vi "login_bage.vi"() -> ()   [LabVIEW 2016]
uses:
  <vilib>/Utility/config.llb/Write Key (String).vi
  <vilib>/Utility/config.llb/Read Key (String).vi
  <vilib>/Utility/file.llb/Write Delimited Spreadsheet (string).vi
  <vilib>/Utility/config.llb/NI_LVConfig.lvlib
panel:
  in  "Choose the CSV file here":path
  in  "Tab Control":enum32{"SIGN IN", "SIGN UP"}(tab)
  in  "Cluster":T1
  in  "Cluster 2":T2
  in  "Choose the INI  file here":path
  out "WARNING":bool
  out "number":dbl[](array[numeric])
  out "Array":string[](array[string])
  # "LOGIN PAGE"
  # "SIGN IN"
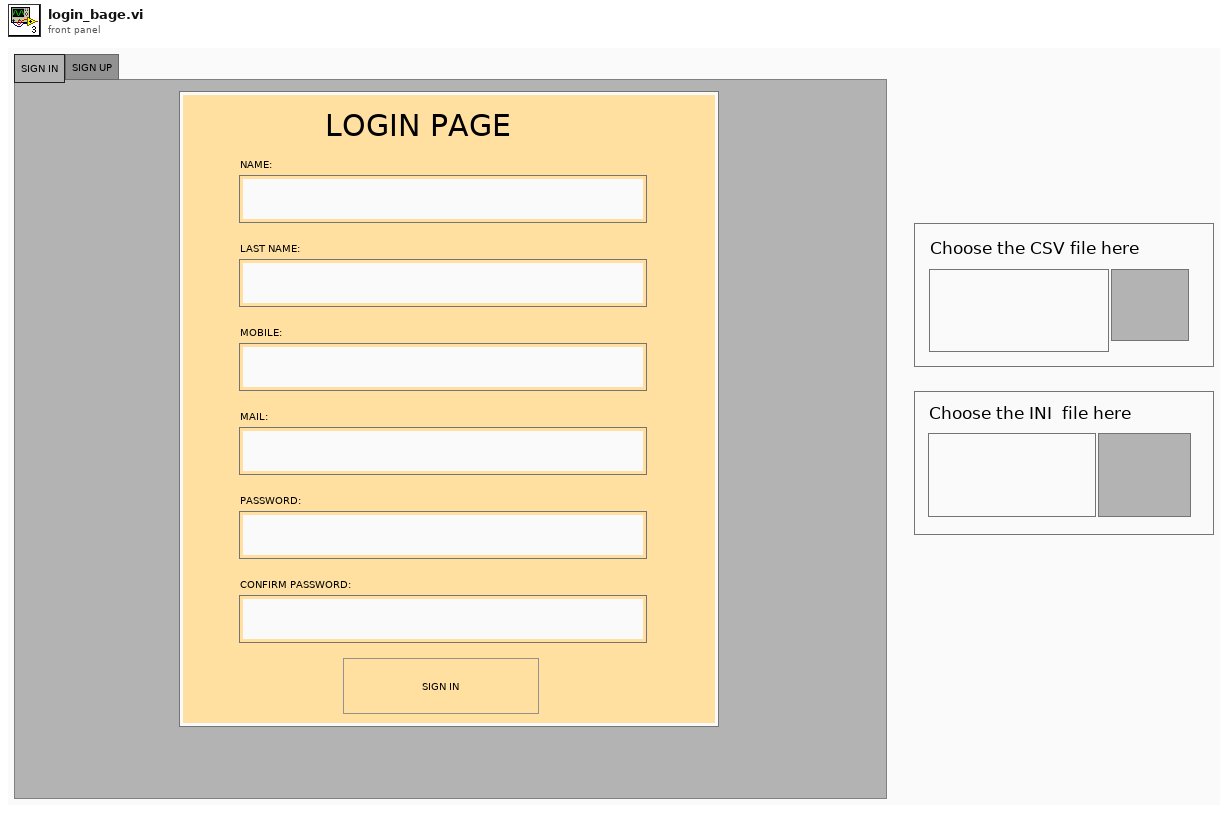
[diagram p1: front panel]
types:
  T1 = cluster{"NAME:":string, "LAST NAME:":string, "MOBILE:":string, "MAIL: ":string, "Boolean":bool, "PASSWORD:":string, "CONFIRM PASSWORD:":string}
  T2 = cluster{"USER NAME:":string, "PASSWORD:":string, "sign":bool}
  T3 = typedef "NI_LVConfig.lvlib/Config Data RefNum.ctl" = refnum<k1>
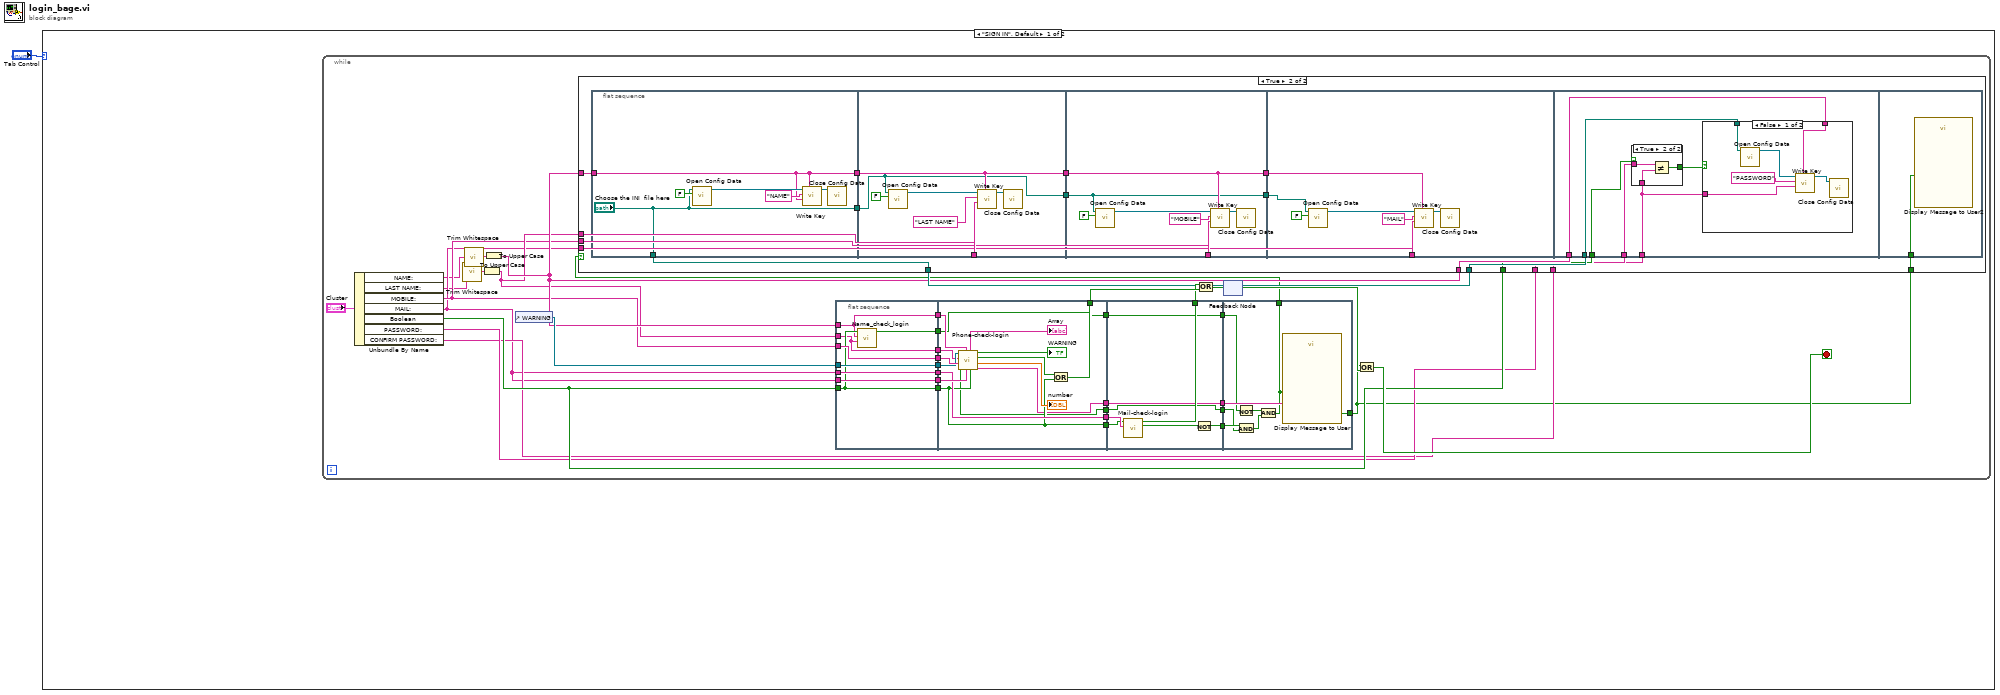
[diagram p0: block diagram]
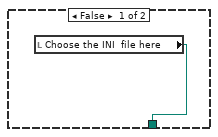
[diagram p2: hidden frame]
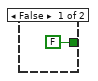
[diagram p3: hidden frame]
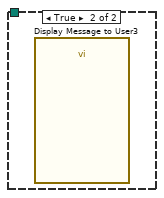
[diagram p4: hidden frame]
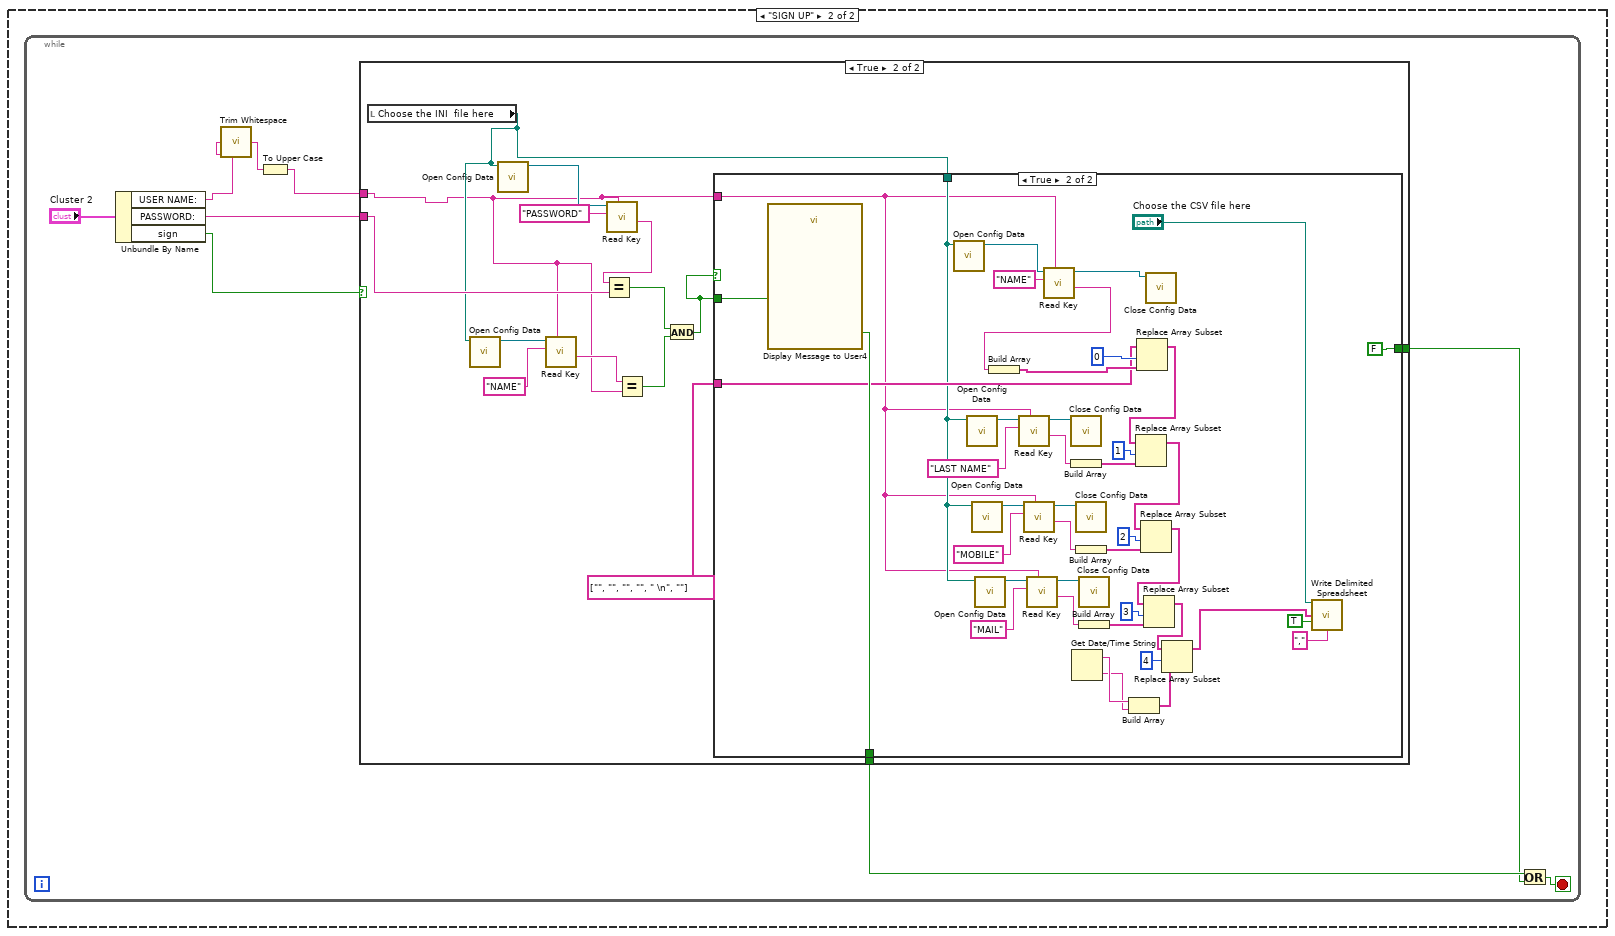
[diagram p5: hidden frame]
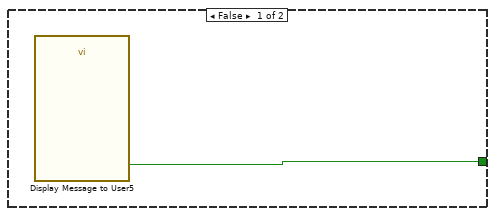
[diagram p7: hidden frame]
diagram:
  n1 = case shown="\"SIGN IN\", Default" "Tab Control" {
    frame "SIGN IN", Default {
      n2 = while {
        stop <- w17 stop-if-true
        n3 = Unbundle By Name("Cluster") -> ("NAME:"=w6:string, "LAST NAME:"=w4:string, "MOBILE:"=w9:string, "MAIL:"=w8:string, "Boolean"=w14:bool, "PASSWORD:"=w13:string, "CONFIRM PASSWORD:"=w12:string)
        n4 = call <vilib>:"Trim Whitespace.vi"("string"=w4) -> ("trimmed string"=w3:string)  [unwired: 1 in]
        n5 = call <vilib>:"Trim Whitespace.vi"("string"=w6) -> ("trimmed string"=w5:string)  [unwired: 1 in]
        n6 = To Upper Case(1:w3) -> (0:w10:string)
        n7 = To Upper Case(1:w5) -> (0:w11:string)
        n8 = control-ref of="WARNING"() -> (w38:refnum<vi>)
        n9 = flat-sequence {
          tunnel: w8 -> [w106]
          tunnel: w38 -> [w107]
          tunnel: w14 -> [w105]
          tunnel: w8 -> [w108]
          tunnel: w9 -> [w109]
          tunnel: w10 -> [w103]
          tunnel: w11 -> [w104]
          tunnel: [w104] -> w28
          tunnel: [w103] -> w27
          tunnel: [w109] -> w26
          tunnel: [w108] -> w25
          tunnel: [w105] -> w24
          tunnel: [w107] -> w23
          tunnel: [w106] -> w22
          tunnel: [w102] -> w21
          tunnel: [w117] -> w36
          tunnel: [w116] -> w37
          tunnel: [w115] -> w34
          tunnel: [w114] -> w33
          tunnel: [w113] -> w32
          tunnel: w28 -> [w112]
          tunnel: w27 -> [w111]
          tunnel: w26 -> [w124]
          tunnel: w25 -> [w123]
          tunnel: w24 -> [w115]
          tunnel: w23 -> [w121]
          tunnel: w22 -> [w116]
          tunnel: w21 -> [w110]
          tunnel: [w110] -> w20
          tunnel: w37 -> [w132]
          tunnel: [w131] -> w35
          tunnel: w34 -> [w126]
          tunnel: [w130] -> w31
          tunnel: w33 -> [w130]
          tunnel: [w129] -> w30
          tunnel: w32 -> [w129]
          tunnel: [w127] -> w29
          tunnel: w20 -> [w125]
          tunnel: [w125] -> w19
          tunnel: w31 -> [w137]
          tunnel: w30 -> [w136]
          tunnel: w29 -> [w138]
          tunnel: w19 -> [w135]
          tunnel: [w134] -> w7
          tunnel: [w133] -> w2
          frame #0 {
            n10 = call "Name_check_login.vi"("LAST NAME:"=w103, "NAME:"=w104, "Boolean"=w105) -> ("OK"=w102:bool)  [unwired: 8 in]
          }
          frame #1 {
            n11 = call "Phone-check-login.vi"("Boolean"=w115, "MAIL:"=w123, "NAME:"=w112, "MOBILE:"=w124, "LAST NAME:"=w111, "Boolean in"=w121) -> ("Info_data"=w113:string, "number"=→"number":dbl[], "Boolean 2"=w122:bool, "WARNING"=→"WARNING":bool, "Array"=→"Array":string[], "sts"=w114:bool)
            n12 = Or(x=w122, y=w115) -> (x .or. y?=w117:bool)
          }
          frame #2 {
            n13 = call "Mail-check-login.vi"("MAIL:"=w132, "Boolean"=w126) -> ("OK2"=w128:bool, "OK"=w131:bool)  [unwired: 8 in]
            n14 = Not(x=w128) -> (.not. x?=w127:bool)
          }
          frame #3 {
            n15 = Not(x=w135) -> (.not. x?=w140:bool)
            n16 = And(x=w138, y=w137) -> (x .and. y?=w139:bool)
            n17 = And(x=w140, y=w139) -> (x .and. y?=w133:bool)
            n18 = call "Display Message to User"("Enable"=w133, "Message"=w136) -> ("OK"=w134:bool)  [unwired: 8 in, 1 out]
          }
        }
        n19 = Or(x=w35, y=w36) -> (x .or. y?=w18:bool)
        n20 = feedback #1() -> (w15:path)  [unwired: 1 in]
        n21 = case shown="True" w2 {
          tunnel: w11 -> [_ w57]
          tunnel: w10 -> [_ w53]
          tunnel: w9 -> [_ w52]
          tunnel: w8 -> [_ w51]
          tunnel: [w40 w47] -> w16
          tunnel: w15 -> [_ w46]
          tunnel: w11 -> [_ w45]
          tunnel: w14 -> [_ w44]
          tunnel: w13 -> [_ w43]
          tunnel: w12 -> [_ w42]
          tunnel: w7 -> [_ w41]
          frame False {
            n22 = local read "Choose the INI  file here"() -> (w40:path)
          }
          frame True {
            n23 = flat-sequence {
              tunnel: w57 -> [w58]
              tunnel: [w58] -> w56
              tunnel: ["Choose the INI  file here"] -> w50
              tunnel: ["Choose the INI  file here"] -> w47
              tunnel: w56 -> [w69]
              tunnel: [w69] -> w55
              tunnel: w53 -> [w64]
              tunnel: w50 -> [w65]
              tunnel: [w65] -> w49
              tunnel: w55 -> [w76]
              tunnel: [w76] -> w54
              tunnel: w52 -> [w71]
              tunnel: w49 -> [w72]
              tunnel: [w72] -> w48
              tunnel: w54 -> [w82]
              tunnel: w51 -> [w78]
              tunnel: w48 -> [w79]
              tunnel: w46 -> [w90]
              tunnel: w45 -> [w89]
              tunnel: w44 -> [w88]
              tunnel: w43 -> [w87]
              tunnel: w42 -> [w86]
              tunnel: w41 -> [w101]
              frame #0 {
                n24 = call <vilib>:"Open Config Data.vi"("create file if necessary (T)"=FALSE, "configuration file path"="Choose the INI  file here") -> ("refnum"=w60:T3)  [unwired: 7 in, 2 out]
                n25 = call-poly <vilib>:"Write Key.vi"("section"=w58, "value"=w58, "key"="NAME", "refnum"=w60) -> ("refnum out"=w62:T3)  [unwired: 5 in, 2 out]
                n26 = call <vilib>:"Close Config Data.vi"("refnum"=w62) -> ()  [unwired: 9 in, 2 out]
              }
              frame #1 {
                n27 = call <vilib>:"Open Config Data.vi"("create file if necessary (T)"=FALSE, "configuration file path"=w65) -> ("refnum"=w66:T3)  [unwired: 7 in, 2 out]
                n28 = call-poly <vilib>:"Write Key.vi"("section"=w69, "value"=w64, "key"="LAST NAME", "refnum"=w66) -> ("refnum out"=w68:T3)  [unwired: 5 in, 2 out]
                n29 = call <vilib>:"Close Config Data.vi"("refnum"=w68) -> ()  [unwired: 9 in, 2 out]
              }
              frame #2 {
                n30 = call <vilib>:"Open Config Data.vi"("create file if necessary (T)"=FALSE, "configuration file path"=w72) -> ("refnum"=w73:T3)  [unwired: 7 in, 2 out]
                n31 = call-poly <vilib>:"Write Key.vi"("section"=w76, "value"=w71, "key"="MOBILE", "refnum"=w73) -> ("refnum out"=w75:T3)  [unwired: 5 in, 2 out]
                n32 = call <vilib>:"Close Config Data.vi"("refnum"=w75) -> ()  [unwired: 9 in, 2 out]
              }
              frame #3 {
                n33 = call <vilib>:"Open Config Data.vi"("create file if necessary (T)"=FALSE, "configuration file path"=w79) -> ("refnum"=w80:T3)  [unwired: 7 in, 2 out]
                n34 = call-poly <vilib>:"Write Key.vi"("section"=w82, "value"=w78, "key"="MAIL", "refnum"=w80) -> ("refnum out"=w84:T3)  [unwired: 5 in, 2 out]
                n35 = call <vilib>:"Close Config Data.vi"("refnum"=w84) -> ()  [unwired: 9 in, 2 out]
              }
              frame #4 {
                n36 = case shown="True" w88 {
                  tunnel: w87 -> [_ w94]
                  tunnel: [FALSE w93] -> w85
                  tunnel: w86 -> [_ w92]
                  frame False {
                  }
                  frame True {
                    n37 = Not Equal?(x=w94, y=w92) -> (x != y?=w93:bool)
                  }
                }
                n38 = case shown="False" w85 {
                  tunnel: w90 -> [w100 _]
                  tunnel: w86 -> [w97 _]
                  tunnel: w89 -> [w95 _]
                  frame False {
                    n39 = call <vilib>:"Open Config Data.vi"("configuration file path"=w100) -> ("refnum"=w99:T3)  [unwired: 8 in, 2 out]
                    n40 = call-poly <vilib>:"Write Key.vi"("section"=w95, "value"=w97, "key"="PASSWORD", "refnum"=w99) -> ("refnum out"=w96:T3)  [unwired: 5 in, 2 out]
                    n41 = call <vilib>:"Close Config Data.vi"("refnum"=w96) -> ()  [unwired: 9 in, 2 out]
                  }
                  frame True {
                    n42 = call "Display Message to User3"() -> ()  [unwired: 10 in, 2 out]
                  }
                }
              }
              frame #5 {
                n43 = call "Display Message to User2"("Enable"=w101) -> ()  [unwired: 9 in, 2 out]
              }
            }
          }
        }
        n44 = feedback-in #1(w16) -> ()
        n45 = Or(x=w7, y=w18) -> (x .or. y?=w17:bool)
      }
    }
    frame "SIGN UP" {
      n46 = while {
        stop <- w148 stop-if-true
        n47 = Unbundle By Name("Cluster 2") -> ("USER NAME:"=w142:string, "PASSWORD:"=w144:string, "sign"=w149:bool)
        n48 = call <vilib>:"Trim Whitespace.vi"("string"=w142) -> ("trimmed string"=w141:string)  [unwired: 1 in]
        n49 = To Upper Case(1:w141) -> (0:w145:string)
        n50 = case shown="True" w149 {
          tunnel: w145 -> [_ w150]
          tunnel: w144 -> [_ w162]
          tunnel: [_ w160] -> w147
          tunnel: [_ w159] -> w146
          frame False {
          }
          frame True {
            n51 = local read "Choose the INI  file here"() -> (w156:path)
            n52 = call <vilib>:"Open Config Data.vi"("configuration file path"=w156) -> ("refnum"=w157:T3)  [unwired: 8 in, 2 out]
            n53 = call <vilib>:"Open Config Data.vi"("configuration file path"=w156) -> ("refnum"=w164:T3)  [unwired: 8 in, 2 out]
            n54 = call-poly <vilib>:"Read Key.vi"("section"=w150, "key"="NAME", "refnum"=w157) -> ("value"=w154:string)  [unwired: 5 in, 3 out]
            n55 = call-poly <vilib>:"Read Key.vi"("section"=w150, "key"="PASSWORD", "refnum"=w164) -> ("value"=w161:string)  [unwired: 5 in, 3 out]
            n56 = Equal?(x=w161, y=w162) -> (x = y?=w152:bool)
            n57 = Equal?(x=w154, y=w150) -> (x = y?=w151:bool)
            n58 = And(x=w152, y=w151) -> (x .and. y?=w153:bool)
            n59 = case shown="True" w153 {
              tunnel: w153 -> [_ w207]
              tunnel: [_ w206] -> w160
              tunnel: [w165 FALSE ("OK")] -> w159
              tunnel: w156 -> [_ w175]
              tunnel: string[] ["", "", "", "", " \n", ""] -> [_ w198]
              tunnel: w150 -> [_ w169]
              frame False {
                n60 = call "Display Message to User5"() -> ("OK"=w165:bool)  [unwired: 10 in, 1 out]
              }
              frame True {
                n61 = call "Display Message to User4"("Enable"=w207) -> ("OK"=w206:bool)  [unwired: 9 in, 1 out]
                n62 = call <vilib>:"Open Config Data.vi"("configuration file path"=w175) -> ("refnum"=w203:T3)  [unwired: 8 in, 2 out]
                n63 = call <vilib>:"Open Config Data.vi"("configuration file path"=w175) -> ("refnum"=w195:T3)  [unwired: 8 in, 2 out]
                n64 = call <vilib>:"Open Config Data.vi"("configuration file path"=w175) -> ("refnum"=w183:T3)  [unwired: 8 in, 2 out]
                n65 = call <vilib>:"Open Config Data.vi"("configuration file path"=w175) -> ("refnum"=w174:T3)  [unwired: 8 in, 2 out]
                n66 = call-poly <vilib>:"Read Key.vi"("section"=w169, "key"="LAST NAME", "refnum"=w195) -> ("value"=w192:string, "refnum out"=w197:T3)  [unwired: 5 in, 2 out]
                n67 = call-poly <vilib>:"Read Key.vi"("section"=w169, "key"="MOBILE", "refnum"=w183) -> ("value"=w186:string, "refnum out"=w181:T3)  [unwired: 5 in, 2 out]
                n68 = call-poly <vilib>:"Read Key.vi"("section"=w169, "key"="MAIL", "refnum"=w174) -> ("value"=w176:string, "refnum out"=w173:T3)  [unwired: 5 in, 2 out]
                n69 = call-poly <vilib>:"Read Key.vi"("section"=w169, "key"="NAME", "refnum"=w203) -> ("value"=w199:string, "refnum out"=w202:T3)  [unwired: 5 in, 2 out]
                n70 = Build Array(w199) -> (w200:string[])
                n71 = call <vilib>:"Close Config Data.vi"("refnum"=w197) -> ()  [unwired: 9 in, 2 out]
                n72 = Build Array(w192) -> (w194:string[])
                n73 = Get Date/Time String() -> (date string=w168:string, time string=w167:string)  [unwired: 3 in]
                n74 = call <vilib>:"Close Config Data.vi"("refnum"=w181) -> ()  [unwired: 9 in, 2 out]
                n75 = Build Array(w186) -> (w184:string[])
                n76 = call <vilib>:"Close Config Data.vi"("refnum"=w173) -> ()  [unwired: 9 in, 2 out]
                n77 = Build Array(w176) -> (w178:string[])
                n78 = Build Array(w168, w167) -> (w166:string[])
                n79 = Replace Array Subset(array=w198, new element=w200, index=0) -> (w191:string[])
                n80 = Replace Array Subset(array=w191, new element=w194, index=1) -> (w180:string[])
                n81 = Replace Array Subset(array=w180, new element=w184, index=2) -> (w172:string[])
                n82 = Replace Array Subset(array=w172, new element=w178, index=3) -> (w171:string[])
                n83 = call <vilib>:"Close Config Data.vi"("refnum"=w202) -> ()  [unwired: 9 in, 2 out]
                n84 = Replace Array Subset(array=w171, new element=w166, index=4) -> (w187:string[])
                n85 = call-poly <vilib>:"Write Delimited Spreadsheet.vi"("file path (dialog if empty)"="Choose the CSV file here", "1D data"=w187, "append to file? (new file:F)"=TRUE, "delimiter (\\t)"="," ("delimiter (\\t)")) -> ()  [unwired: 10 in, 2 out]
              }
            }
          }
        }
        n86 = Or(x=w147, y=w146) -> (x .or. y?=w148:bool)
      }
    }
  }
